vi "ROI entry screen-LBox edit cells_030220.vi"(8 "error in (no error)":errorcluster, 11 "Selected Cell":T1) -> (0 "error out":errorcluster)   [LabVIEW 2020]
uses:
  <vilib>/Utility/miscctls.llb/LVRowAndColumnTypeDef.ctl
  Typedefs/ROI management FG states.ctl
  Globals/gl_ROI Entry UI globals.vi
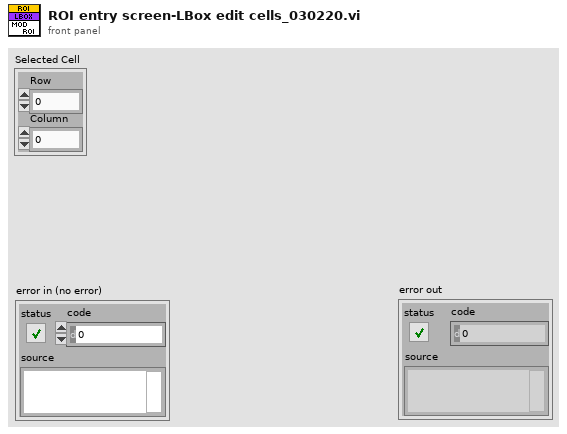
[diagram p1: front panel]
types:
  T1 = typedef "LVRowAndColumnTypeDef.ctl" = cluster{"Row":i32, "Column":i32}
  T2 = typedef "ROI management FG states.ctl" = enum16{"Read", "Write", "Write-from dataset", "Clear Last", "Clear All", "Delete ROI", "Update ROIs time", "Reload last ROI set", "Modify ROI Parameters", "Offset all ROI", "Offset visible ROI", "Modify Dwell Time", "Modify Laser Power"}
  T3 = typedef "ROI entry screen ctrl refs cluster.ctl" = cluster{"Done button":refnum<vi>, "Imaging button":refnum<vi>, "Acquisition button":refnum<vi>, "Scan dwell time per pixel (us)":refnum<vi>, "# of planes":refnum<vi>, "Zoom Ctrl":refnum<vi>, "Equal size":refnum<vi>, "Channel":refnum<vi>, "Image Display":refnum<vi>, "Z-Plane Selector":refnum<vi>, "Number of lines left":refnum<vi>, "Z-stack folder path":refnum<vi>, "POI Density":refnum<vi>, "Arb Plane Entry":refnum<vi>, "Whole Plane":refnum<vi>, "Line Mode":refnum<vi>, "Clear Last":refnum<vi>, "Clear All":refnum<vi>, "Delete Lines":refnum<vi>, "Trial Length (sec)":refnum<vi>, "Palette Type":refnum<vi>, "Intensity slider":refnum<vi>, "# POI":refnum<vi>, "Max Z Proj":refnum<vi>, "Zplane ind":refnum<vi>, "Wavelength (nm)":refnum<vi>, "Number of Trials":refnum<vi>, "Funct stim.trig.enable":refnum<vi>, "Funct stim.trig.delay (s)":refnum<vi>, "Line Mode":refnum<vi>, "Step size (µm)":refnum<vi>, "ROI move mode":refnum<vi>, "Cool-down time (s)":refnum<vi>, "Enable cool-down time":refnum<vi>, "Motor Z ind. (um)":refnum<vi>, "AOL Z ind. (um)":refnum<vi>, "Load Reference Image":refnum<vi>, "Rel.  Res.":refnum<vi>, "ROI LIST":refnum<vi>, "Show All":refnum<vi>, "ROI Type":refnum<vi>, "Start Plane":refnum<vi>, "Stop Plane":refnum<vi>, "Offset ROI":refnum<vi>, "Tab Control":refnum<vi>, "Laser Power(%)":refnum<vi>, "Cycle rate":refnum<vi>, "FOV (Ind.)":refnum<vi>, "Frame Size (Ind.)":refnum<vi>, "Resolution (Ind.)":refnum<vi>, "Pixel Density (Ind)":refnum<vi>, "Laser Power (Ind.)":refnum<vi>, "Dwell Time (Ind.)":refnum<vi>, "Adj MC":refnum<vi>}
  T4 = typedef "ROI parameters data type.ctl" = cluster{"ROI index":dbl, "ROI ID":dbl, "ROI Time (ns)":dbl, "Pixels in ROI":dbl, "X start":dbl, "Y start":dbl, "Z start":dbl, "X stop":dbl, "Y stop":dbl, "Z stop":dbl, "Angle (deg)":dbl, "Composite ID":dbl, "Number of lines":dbl, "Frame Size":dbl, "Zoom":dbl, "Laser Power (%)":dbl, "ROI group ID":dbl, "Resolution":dbl, "Dwell Time per pixel":dbl, "Pixels per miniscan":dbl, "Original FOV (um)":dbl, "Apparent Frame Size":dbl, "Z Plane Idx":i32[], "Z Plane codes":i32[]}
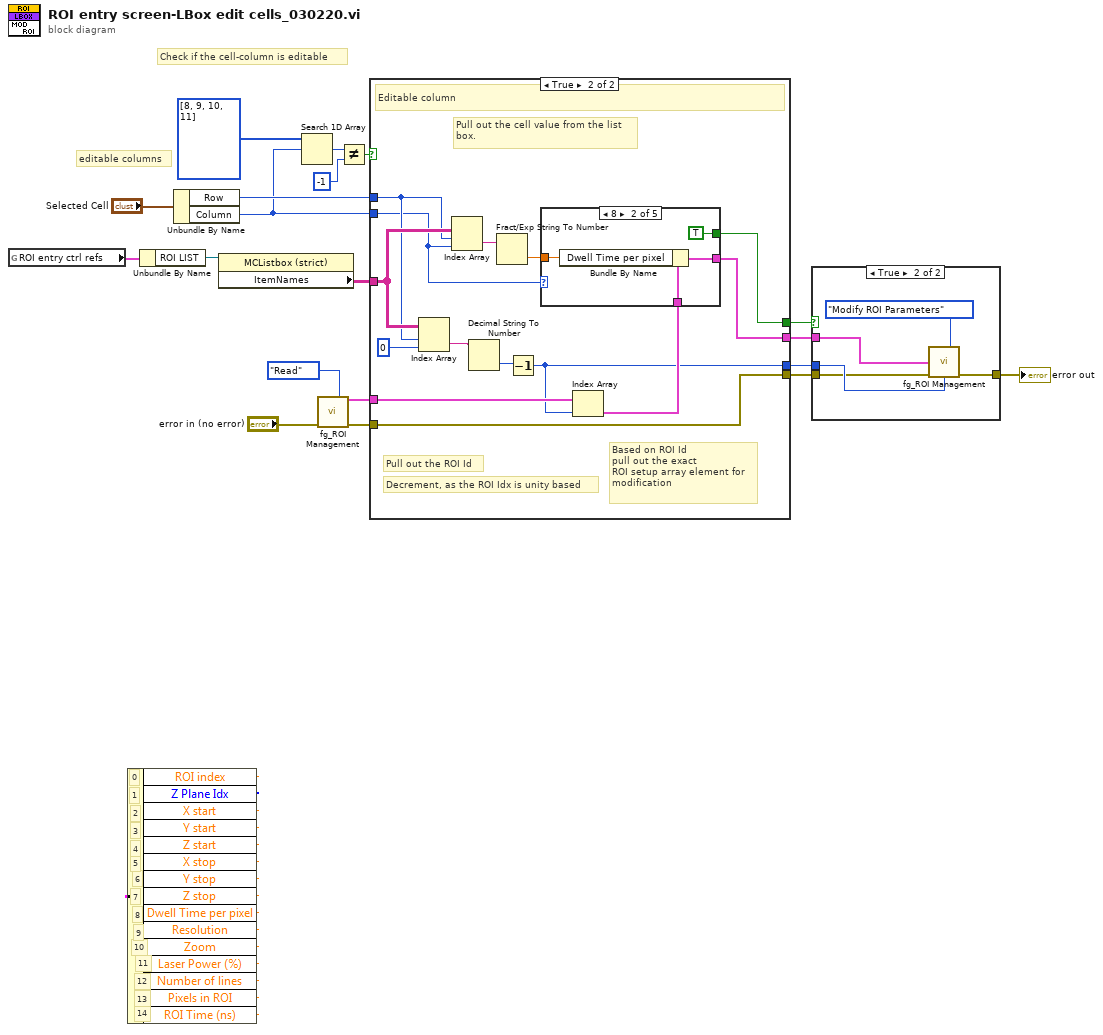
[diagram p0: block diagram]
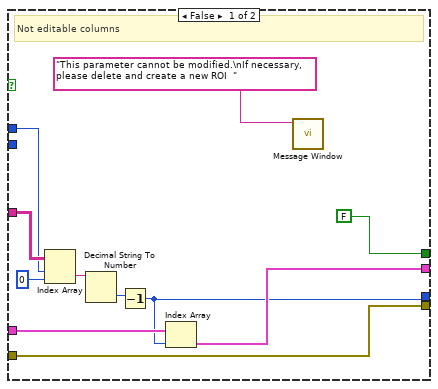
[diagram p3: hidden frame]
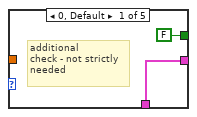
[diagram p4: hidden frame]
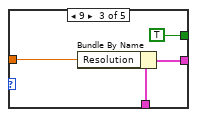
[diagram p5: hidden frame]
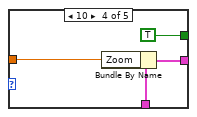
[diagram p6: hidden frame]
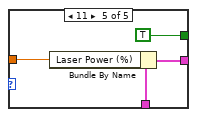
[diagram p7: hidden frame]
diagram:
  # "editable columns"
  # "Check if the cell-column is editable"
  # "14"
  # "13"
  # "12"
  # "11"
  # "10"
  # "9"
  # "8"
  # "7"
  # "6"
  # "5"
  # "4"
  # "3"
  # "2"
  # "1"
  # "0"
  n1 = global read "gl_ROI Entry UI globals.vi" "ROI entry ctrl refs"() -> (w15:T3)
  n2 = Unbundle By Name(w15) -> ("ROI LIST"=w12:refnum<vi>)
  n3 = Unbundle By Name("Selected Cell") -> ("Row"=w10:i32, "Column"=w4:i32)
  n4 = property class="MCListbox (strict)"(reference=w12) -> ("ItemNames"=w11:string[][])  [unwired: 1 in, 2 out]
  n5 = Search 1D Array(1D array=i32[] [8, 9, 10, 11], element=w4) -> (index of element=w6:i32)  [unwired: 1 in]
  n6 = call "fg_ROI Management.vi"("Function"=ROI_management_FG_states."Read", "error in (no error)"="error in (no error)") -> ("ROI Setup"=w17:T4[], "error out"=w13:errorcluster)  [unwired: 7 in, 5 out]
  n7 = Not Equal?(x=w6, y=-1) -> (x != y?=w3:bool)
  n8 = case shown="True" w3 {
    tunnel: w17 -> [w25 w39]
    tunnel: [FALSE w32] -> w16
    tunnel: w13 -> [w21 w31]
    tunnel: w11 -> [w24 w44]
    tunnel: w10 -> [w23 w43]
    tunnel: [w22 w35] -> w9
    tunnel: [w20 w34] -> w8
    tunnel: w4 -> [_ w33]
    tunnel: [w21 w31] -> w2
    frame False {
      # "Not editable columns"
      n9 = Index Array(array=w24, index (row)=w23, index (col)=0 ("disabled index (col)")) -> (element=w27:string)
      n10 = Decimal String To Number(string=w27) -> (number=w26:i32)  [unwired: 2 in, 1 out]
      n11 = Decrement(x=w26) -> (x-1=w20:i32)
      n12 = Index Array(array=w25, index=w20) -> (element=w22:T4)
      n13 = call "Message Window.vi"("Message string"="This parameter cannot be modified.\nIf necessary, please delete and create a new ROI  ") -> ()  [unwired: 10 in, 1 out]
    }
    frame True {
      # "Decrement, as the ROI Idx is unity based"
      # "Based on ROI Id \npull out the exact\nROI setup array element for\nmodification"
      # "Pull out the ROI Id"
      # "Pull out the cell value from the list\nbox."
      # "Editable column"
      n14 = Index Array(array=w44, index (row)=w43, index (col)=0 ("disabled index (col)")) -> (element=w41:string)
      n15 = Index Array(array=w44, index (row)=w43, index (col)=w33) -> (element=w37:string)
      n16 = Decimal String To Number(string=w41) -> (number=w40:i32)  [unwired: 2 in, 1 out]
      n17 = Fract/Exp String To Number(string=w37) -> (number=w36:dbl)  [unwired: 3 in, 1 out]
      n18 = Decrement(x=w40) -> (x-1=w34:i32)
      n19 = Index Array(array=w39, index=w34) -> (element=w38:T4)
      n20 = case shown="8" w33 {
        tunnel: w38 -> [w46 w50 w54 w58 w62]
        tunnel: w36 -> [_ w49 w53 w57 w61]
        tunnel: [w46 w48 w52 w56 w60] -> w35
        tunnel: [FALSE TRUE TRUE TRUE TRUE] -> w32
        frame 0, Default {
          # "additional\ncheck - not strictly\nneeded"
        }
        frame 8 {
          n21 = Bundle By Name(cluster=w50, "Dwell Time per pixel"=w49) -> (w48:T4)
        }
        frame 9 {
          n22 = Bundle By Name(cluster=w54, "Resolution"=w53) -> (w52:T4)
        }
        frame 10 {
          n23 = Bundle By Name(cluster=w58, "Zoom"=w57) -> (w56:T4)
        }
        frame 11 {
          n24 = Bundle By Name(cluster=w62, "Laser Power (%)"=w61) -> (w60:T4)
        }
      }
    }
  }
  n25 = case shown="True" w16 {
    tunnel: w9 -> [_ w67]
    tunnel: w8 -> [_ w66]
    tunnel: w2 -> [w63 w65]
    tunnel: [w63 w64] -> w1
    frame False {
    }
    frame True {
      n26 = call "fg_ROI Management.vi"("Function"=ROI_management_FG_states."Modify ROI Parameters", "XYZ"=w67, "error in (no error)"=w65, "ROI Setup Array Idx to modify"=w66) -> ("error out"=w64:errorcluster)  [unwired: 5 in, 6 out]
    }
  }
  "error out" <- w1
